vi "clone.vi"(0 "reference":refnum<class "ImplicitParameterNode.lvclass">, 5 "error in (no error)":errorcluster) -> (14 "reference out":refnum<class "ImplicitParameterNode.lvclass">, 15 "clonedNode":refnum<class "AbstractNode.lvclass">, 19 "error out":errorcluster)   [LabVIEW 2016, in "ImplicitParameterNode.lvclass"]
doc: "public Object clone()"
uses:
  <resource>/Framework/Providers/Open_GDS/UML/ImplicitParameterNode_class/ImplicitParameterNode.lvclass
  C:/Program Files (x86)/National Instruments/LabVIEW 2016/resource/Framework/Providers/Open_GDS/UML/AbstractNode_class/AbstractNode.lvclass
  <resource>/Framework/Providers/Open_GDS/UML/AbstractNode_class/AbstractNode.lvclass
  <resource>/Framework/Providers/Open_GDS/UML/MultiLineString_class/MultiLineString.lvclass
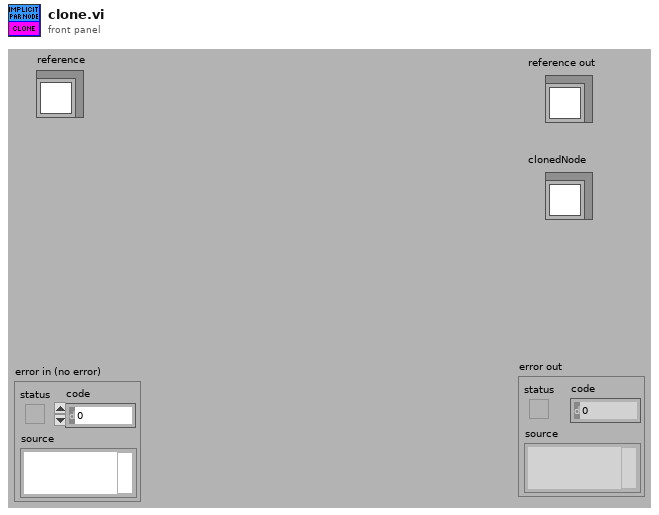
[diagram p1: front panel]
types:
  T1 = typedef "ImplicitParameterNode.lvclass/ObjectAttributes.ctl" = cluster{"topHeight":dbl, "name":refnum<class "MultiLineString.lvclass">, "DEFAULT_TOP_HEIGHT":i32, "DEFAULT_WIDTH":i32, "DEFAULT_HEIGHT":i32}
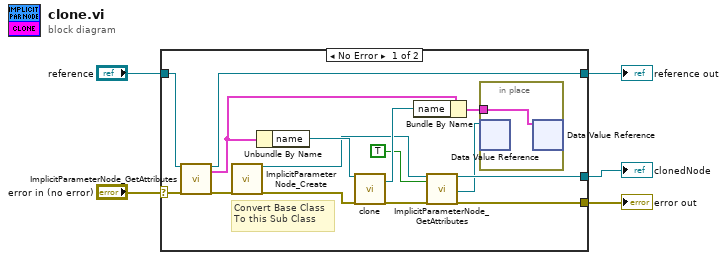
[diagram p0: block diagram]
diagram:
  n1 = case shown="No Error" "error in (no error)" {
    selector: "error in (no error)" -> [w19 w22]
    tunnel: "reference" -> [w20 w23]
    tunnel: [w8 w22] -> w4
    tunnel: [w12 w23] -> w3
    tunnel: [w9 _] -> w1
    frame No Error {
      # "Convert Base Class\nTo this Sub Class"
      n2 = call <resource>:"ImplicitParameterNode_GetAttributes.vi"("reference in"=w20, "error in (no error)"=w19) -> ("reference out"=w12:refnum<class "ImplicitParameterNode.lvclass">, "Data"=w10:T1, "error out"=w14:errorcluster)  [unwired: 1 in, 14 out]
      n3 = call <resource>:"ImplicitParameterNode_Create.vi"("error in (no error)"=w14) -> ("reference out"=w13:refnum<class "ImplicitParameterNode.lvclass">, "error out"=w18:errorcluster)  [unwired: 17 in]
      n4 = Unbundle By Name(w10) -> ("name"=w17:refnum<class "MultiLineString.lvclass">)
      n5 = call-dynamic "clone.vi"("reference"=w17, "error in (no error)"=w18) -> ("clonedMultiLineString"=w15:refnum<class "MultiLineString.lvclass">, "error out"=w16:errorcluster)  [unwired: 15 in, 1 out]
      n6 = Bundle By Name(cluster=w10, "name"=w15) -> (w6:T1)
      n7 = call <resource>:"ImplicitParameterNode_GetAttributes.vi"("reference in"=w13, "OnlyGetDvrReference(False)"=TRUE, "error in (no error)"=w16) -> ("reference out"=w9:refnum<class "ImplicitParameterNode.lvclass">, "DataRef"=w7:refnum<data-value>, "error out"=w8:errorcluster)  [unwired: 13 in, 1 out]
      n8 = in-place {
        in-place-border: w6 -> [w21]
        n9 = in-place-dvr #1(w7) -> ()  [unwired: 2 out]
        n10 = in-place-dvr #1(w21) -> ()  [unwired: 2 out]
      }
    }
    frame Error {
    }
  }
  "reference out" <- w3
  "error out" <- w4
  "clonedNode" <- w1
